vi "Calculate 2D meander.vi"(0 "Line orientation (T: vert.)":bool=TRUE, 1 "Direction ax1 (T:+)":bool=TRUE, 2 "Direction ax2 (T:+)":bool=TRUE, 3 "Start position ax1":dbl format="%.6f", 4 "Start position ax2":dbl format="%.6f", 6 "Range ax1":dbl format="%.2f", 7 "Step size":dbl format="%.2f", 8 "Range ax2":dbl format="%.2f") -> (10 "Min. pos. ax2":dbl format="%.6f", 11 "Max. pos. ax2":dbl format="%.6f", 12 "1D pos. array ax2":dbl[](array[numeric]) format="%.6f", 14 "1D pos. array ax1":dbl[](array[numeric]) format="%.6f", 15 "Min. pos. ax1":dbl format="%.6f", 16 "Max. pos. ax1":dbl format="%.6f", 17 "No. of steps":i32, 18 "2D intensity array":dbl[][](array[numeric]) format="%.6f")   [LabVIEW 2026]
doc: "Calculates position values for a 2D linear meander scan and initializes intensity array according to Start position of axes 1 and 2, Step size, range of axes 1 and 2 and scan directions of axes 1 and 2. The VI returns Minimum position, Maximum position, No. of steps and initialized 1D position array for axes 1 and 2 and a 2D intensity array."
panel:
  # "Calculates position values for a 2D linear meander scan and initializes intensity array."
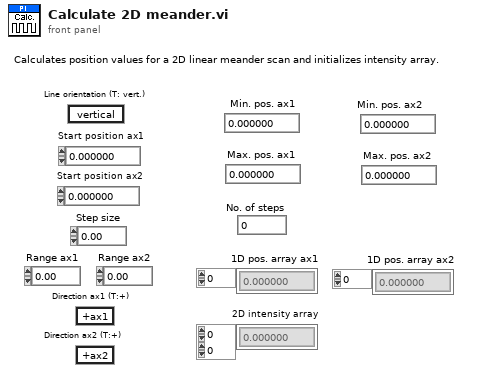
[diagram p1: front panel]
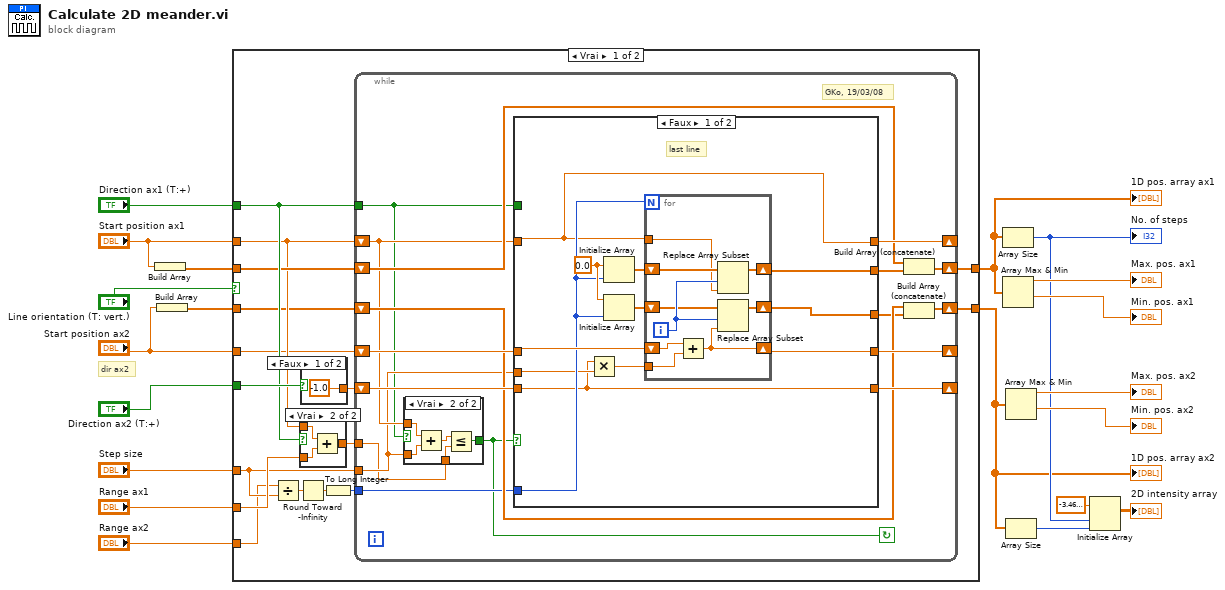
[diagram p0: block diagram]
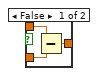
[diagram p2: hidden frame]
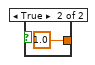
[diagram p3: hidden frame]
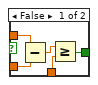
[diagram p4: hidden frame]
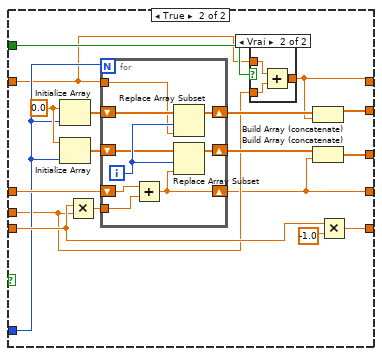
[diagram p5: hidden frame]
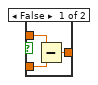
[diagram p6: hidden frame]
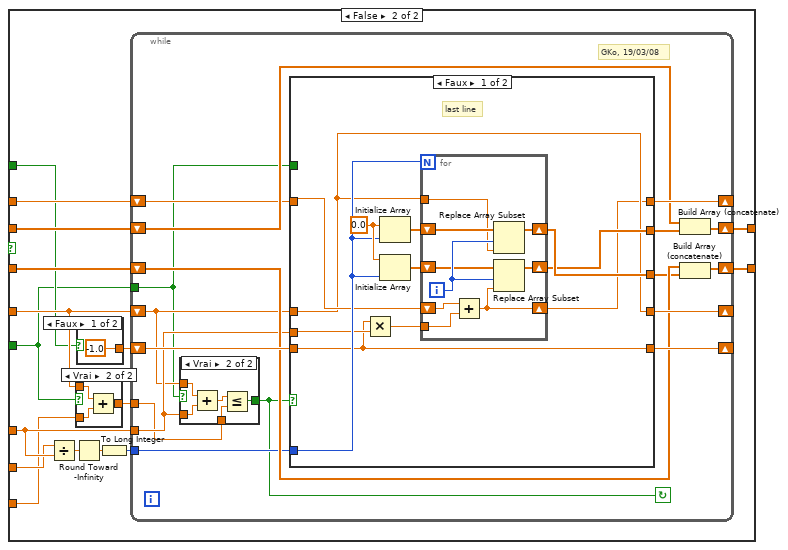
[diagram p7: hidden frame]
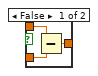
[diagram p8: hidden frame]
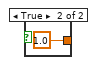
[diagram p9: hidden frame]
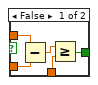
[diagram p10: hidden frame]
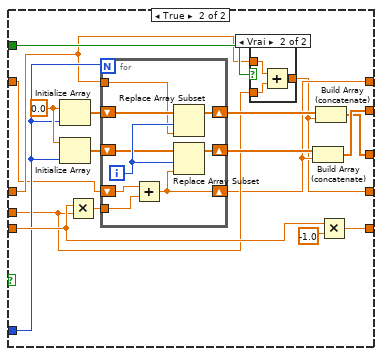
[diagram p11: hidden frame]
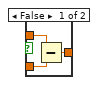
[diagram p12: hidden frame]
diagram:
  # "dir ax2"
  n1 = Build Array("Start position ax1") -> (w7:dbl[])
  n2 = Build Array("Start position ax2") -> (w5:dbl[])
  n3 = case shown="Vrai" "Line orientation (T: vert.)" {
    tunnel: "Direction ax2 (T:+)" -> [w35 w128]
    tunnel: "Range ax1" -> [w33 w127]
    tunnel: "Step size" -> [w32 w139]
    tunnel: "Range ax2" -> [w29 w126]
    tunnel: "Direction ax1 (T:+)" -> [w28 w129]
    tunnel: w7 -> [w26 w135]
    tunnel: "Start position ax1" -> [w25 w134]
    tunnel: w5 -> [w24 w133]
    tunnel: "Start position ax2" -> [w23 w130]
    tunnel: [w22 w132] -> w3
    tunnel: [w21 w131] -> w2
    frame True {
      n4 = Divide(x=w29, y=w32) -> (x/y=w31:dbl)
      n5 = Round Toward -Infinity(1:w31) -> (0:w30:dbl)
      n6 = case shown="Vrai" w28 {
        tunnel: w25 -> [w38 w42]
        tunnel: w33 -> [w39 w41]
        tunnel: [w37 w40] -> w34
        frame False {
          n7 = Subtract(x=w38, y=w39) -> (x-y=w37:dbl)
        }
        frame True {
          n8 = Add(x=w42, y=w41) -> (x+y=w40:dbl)
        }
      }
      n9 = case shown="Faux" w35 {
        tunnel: [-1.0 ("y") 1.0 ("y")] -> w36
        frame False {
        }
        frame True {
        }
      }
      n10 = To Long Integer(number=w30) -> (32bit integer=w27:i32)
      n11 = while {
        shift-left: w26 -> [w56]
        shift-right: [w54] -> w22
        tunnel: w32 -> [w49]
        shift-right: [w57] -> _
        shift-left: w36 -> [w60]
        shift-right: [w53] -> w21
        shift-left: w24 -> [w52]
        shift-right: [w59] -> _
        shift-left: w25 -> [w50]
        shift-right: [w58] -> _
        shift-left: w23 -> [w61]
        tunnel: w34 -> [w47]
        tunnel: w27 -> [w48]
        tunnel: w28 -> [w45]
        stop <- w46 continue-if-true
        # "GKo, 19/03/08"
        n12 = case shown="Vrai" w45 {
          tunnel: w50 -> [w65 w71]
          tunnel: w49 -> [w66 w70]
          tunnel: [w64 w69] -> w46
          tunnel: w47 -> [w62 w67]
          frame False {
            n13 = Subtract(x=w65, y=w66) -> (x-y=w63:dbl)
            n14 = Greater Or Equal?(x=w63, y=w62) -> (x >= y?=w64:bool)
          }
          frame True {
            n15 = Add(x=w71, y=w70) -> (x+y=w68:dbl)
            n16 = Less Or Equal?(x=w68, y=w67) -> (x <= y?=w69:bool)
          }
        }
        n17 = case shown="Faux" w46 {
          tunnel: w50 -> [w72 w93]
          tunnel: w61 -> [w79 w110]
          tunnel: w49 -> [w74 w96]
          tunnel: [w72 w95] -> w59
          tunnel: [w75 w94] -> w58
          tunnel: w60 -> [w73 w109]
          tunnel: [w73 w106] -> w57
          tunnel: [w77 w108] -> w55
          tunnel: [w76 w107] -> w51
          tunnel: w48 -> [w78 w99]
          tunnel: w45 -> [_ w97]
          frame False {
            w83 = 0.0 ("y")
            # "last line"
            n18 = Multiply(x=w73, y=w74) -> (x*y=w82:dbl)
            n19 = Initialize Array(w83, w78) -> (w81:dbl[])
            n20 = Initialize Array(w83, w78) -> (w80:dbl[])
            n21 = for {
              N: w78 -> [_]
              shift-right: [w90] -> w77
              shift-left: w81 -> [w91]
              shift-right: [w88] -> w76
              shift-left: w80 -> [w89]
              tunnel: w72 -> [w84]
              shift-right: [w86] -> w75
              shift-left: w79 -> [w87]
              tunnel: w82 -> [w85]
              i -> [w92]
              n22 = Add(x=w87, y=w85) -> (x+y=w86:dbl)
              n23 = Replace Array Subset(array=w91, new element=w84, index=w92) -> (w90:dbl[])
              n24 = Replace Array Subset(array=w89, new element=w86, index=w92) -> (w88:dbl[])
            }
          }
          frame True {
            w105 = 0.0 ("y")
            n25 = Initialize Array(w105, w99) -> (w102:dbl[])
            n26 = Initialize Array(w105, w99) -> (w101:dbl[])
            n27 = Multiply(x=w109, y=w96) -> (x*y=w104:dbl)
            n28 = for {
              N: w99 -> [_]
              shift-right: [w123] -> w100
              shift-left: w102 -> [w124]
              shift-right: [w121] -> w98
              shift-left: w101 -> [w122]
              tunnel: w93 -> [w118]
              shift-right: [w119] -> w94
              shift-left: w110 -> [w120]
              tunnel: w104 -> [w117]
              i -> [w125]
              n29 = Add(x=w120, y=w117) -> (x+y=w119:dbl)
              n30 = Replace Array Subset(array=w124, new element=w118, index=w125) -> (w123:dbl[])
              n31 = Replace Array Subset(array=w122, new element=w119, index=w125) -> (w121:dbl[])
            }
            n32 = case shown="Vrai" w97 {
              tunnel: w93 -> [w112 w116]
              tunnel: w96 -> [w113 w115]
              tunnel: [w111 w114] -> w95
              frame False {
                n33 = Subtract(x=w112, y=w113) -> (x-y=w111:dbl)
              }
              frame True {
                n34 = Add(x=w116, y=w115) -> (x+y=w114:dbl)
              }
            }
            n35 = Build Array (concatenate)(w100, w95) -> (w108:dbl[])
            n36 = Build Array (concatenate)(w98, w94) -> (w107:dbl[])
            n37 = Multiply(x=w109, y=-1.0) -> (x*y=w106:dbl)
          }
        }
        n38 = Build Array (concatenate)(w56, w55) -> (w54:dbl[])
        n39 = Build Array (concatenate)(w52, w51) -> (w53:dbl[])
      }
    }
    frame False {
      n40 = Divide(x=w127, y=w139) -> (x/y=w138:dbl)
      n41 = Round Toward -Infinity(1:w138) -> (0:w137:dbl)
      n42 = case shown="Vrai" w128 {
        tunnel: w130 -> [w143 w147]
        tunnel: w126 -> [w144 w146]
        tunnel: [w142 w145] -> w140
        frame False {
          n43 = Subtract(x=w143, y=w144) -> (x-y=w142:dbl)
        }
        frame True {
          n44 = Add(x=w147, y=w146) -> (x+y=w145:dbl)
        }
      }
      n45 = case shown="Faux" w129 {
        tunnel: [-1.0 ("y") 1.0 ("y")] -> w141
        frame False {
        }
        frame True {
        }
      }
      n46 = To Long Integer(number=w137) -> (32bit integer=w136:i32)
      n47 = while {
        shift-left: w135 -> [w162]
        shift-right: [w160] -> w132
        tunnel: w139 -> [w155]
        shift-right: [w163] -> _
        shift-left: w141 -> [w166]
        shift-right: [w159] -> w131
        shift-left: w133 -> [w158]
        shift-right: [w165] -> _
        shift-left: w134 -> [w156]
        shift-right: [w164] -> _
        shift-left: w130 -> [w151]
        tunnel: w140 -> [w153]
        tunnel: w136 -> [w154]
        tunnel: w128 -> [w150]
        stop <- w152 continue-if-true
        # "GKo, 19/03/08"
        n48 = case shown="Vrai" w150 {
          tunnel: w151 -> [w170 w176]
          tunnel: w155 -> [w171 w175]
          tunnel: [w169 w174] -> w152
          tunnel: w153 -> [w167 w172]
          frame False {
            n49 = Subtract(x=w170, y=w171) -> (x-y=w168:dbl)
            n50 = Greater Or Equal?(x=w168, y=w167) -> (x >= y?=w169:bool)
          }
          frame True {
            n51 = Add(x=w176, y=w175) -> (x+y=w173:dbl)
            n52 = Less Or Equal?(x=w173, y=w172) -> (x <= y?=w174:bool)
          }
        }
        n53 = case shown="Faux" w152 {
          tunnel: w156 -> [w181 w198]
          tunnel: w151 -> [w178 w203]
          tunnel: w155 -> [w183 w204]
          tunnel: [w177 w200] -> w165
          tunnel: [w178 w199] -> w164
          tunnel: w166 -> [w182 w215]
          tunnel: [w182 w214] -> w163
          tunnel: [w179 w202] -> w161
          tunnel: [w180 w201] -> w157
          tunnel: w154 -> [w184 w207]
          tunnel: w150 -> [_ w205]
          frame False {
            w188 = 0.0 ("y")
            # "last line"
            n54 = Multiply(x=w182, y=w183) -> (x*y=w187:dbl)
            n55 = Initialize Array(w188, w184) -> (w186:dbl[])
            n56 = Initialize Array(w188, w184) -> (w185:dbl[])
            n57 = for {
              N: w184 -> [_]
              shift-right: [w195] -> w180
              shift-left: w186 -> [w196]
              shift-right: [w193] -> w179
              shift-left: w185 -> [w194]
              tunnel: w178 -> [w189]
              shift-right: [w191] -> w177
              shift-left: w181 -> [w192]
              tunnel: w187 -> [w190]
              i -> [w197]
              n58 = Add(x=w192, y=w190) -> (x+y=w191:dbl)
              n59 = Replace Array Subset(array=w196, new element=w189, index=w197) -> (w195:dbl[])
              n60 = Replace Array Subset(array=w194, new element=w191, index=w197) -> (w193:dbl[])
            }
          }
          frame True {
            w213 = 0.0 ("y")
            n61 = Initialize Array(w213, w207) -> (w210:dbl[])
            n62 = Initialize Array(w213, w207) -> (w209:dbl[])
            n63 = Multiply(x=w215, y=w204) -> (x*y=w212:dbl)
            n64 = for {
              N: w207 -> [_]
              shift-right: [w228] -> w208
              shift-left: w210 -> [w229]
              shift-right: [w226] -> w206
              shift-left: w209 -> [w227]
              tunnel: w203 -> [w223]
              shift-right: [w224] -> w200
              shift-left: w198 -> [w225]
              tunnel: w212 -> [w222]
              i -> [w230]
              n65 = Add(x=w225, y=w222) -> (x+y=w224:dbl)
              n66 = Replace Array Subset(array=w229, new element=w223, index=w230) -> (w228:dbl[])
              n67 = Replace Array Subset(array=w227, new element=w224, index=w230) -> (w226:dbl[])
            }
            n68 = case shown="Vrai" w205 {
              tunnel: w203 -> [w217 w221]
              tunnel: w204 -> [w218 w220]
              tunnel: [w216 w219] -> w199
              frame False {
                n69 = Subtract(x=w217, y=w218) -> (x-y=w216:dbl)
              }
              frame True {
                n70 = Add(x=w221, y=w220) -> (x+y=w219:dbl)
              }
            }
            n71 = Build Array (concatenate)(w206, w200) -> (w202:dbl[])
            n72 = Build Array (concatenate)(w208, w199) -> (w201:dbl[])
            n73 = Multiply(x=w215, y=-1.0) -> (x*y=w214:dbl)
          }
        }
        n74 = Build Array (concatenate)(w162, w161) -> (w160:dbl[])
        n75 = Build Array (concatenate)(w158, w157) -> (w159:dbl[])
      }
    }
  }
  "1D pos. array ax1" <- w3
  "1D pos. array ax2" <- w2
  n76 = Array Size(array=w3) -> (size(s)=w14:i32)
  "No. of steps" <- w14
  n77 = Array Max & Min(array=w3) -> (max value=→"Max. pos. ax1":dbl, min value=→"Min. pos. ax1":dbl)  [unwired: 2 out]
  n78 = Array Max & Min(array=w2) -> (max value=→"Max. pos. ax2":dbl, min value=→"Min. pos. ax2":dbl)  [unwired: 2 out]
  n79 = Array Size(array=w2) -> (size(s)=w13:i32)
  n80 = Initialize Array(-3.469446951953614e-18 ("Element Data"), w14, w13) -> (→"2D intensity array":dbl[][])
